vi "SPI Close Channel.vi"(8 "error in (no error)":errorcluster, 11 "handle":u32) -> (0 "error out":errorcluster, 2 "function return":u32, 3 "handle out":u32)   [LabVIEW 2018, in "libMPSSE-SPI.lvlib"]
doc: "FTDI_API FT_STATUS SPI_CloseChannel(FT_HANDLE handle);"
uses:
  PROJEKT/NIKO/Labview/Niko V6_A/FTDI SPI/libMPSSE-SPI.lvlib
  PROJEKT/NIKO/Labview/Niko V6_A/FTDI SPI/dll/libMPSSE.dll
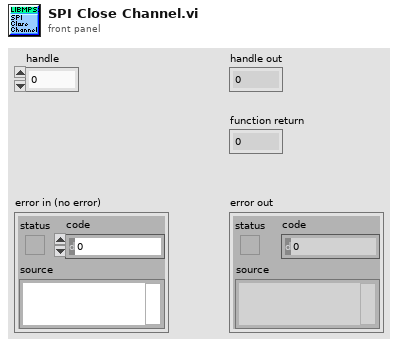
[diagram p1: front panel]
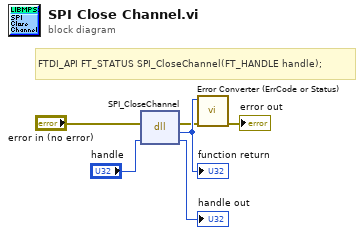
[diagram p0: block diagram]
diagram:
  # "FTDI_API FT_STATUS SPI_CloseChannel(FT_HANDLE handle);"
  n1 = dll-call lib="D:/LABVIEW/PROJEKT/NIKO/Labview/Niko V6_A/FTDI SPI/dll/libMPSSE.*" fn="SPI_CloseChannel"(error in="error in (no error)", "handle"="handle") -> (error out=w2:errorcluster, w6:u32, "handle"=→"handle out":u32)  [unwired: 2 in, 1 out]
  "function return" <- w6
  n2 = call "Error Converter (ErrCode or Status).vi"("error in (no error)"=w2, "error code"=w6) -> ("error out"=→"error out":errorcluster)  [unwired: 9 in]
